vi "Get Result.vi"(8 "error in (no error)":errorcluster, 11 "Addition in":refnum<class "Subtraction.lvclass">) -> (0 "error out":errorcluster, 2 "Result":dbl, 3 "Addition out":refnum<class "Subtraction.lvclass">)   [LabVIEW 2013, in "Operators.lvlib" / "Subtraction.lvclass"]
uses:
  Subtraction.lvclass
  Subtraction.lvclass/Subtraction.ctl
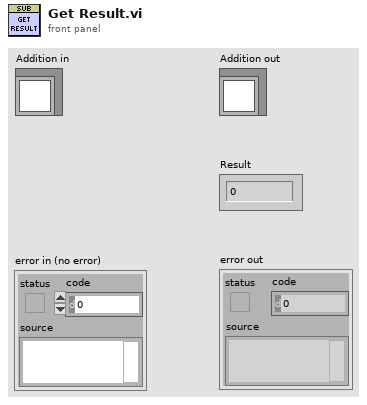
[diagram p1: front panel]
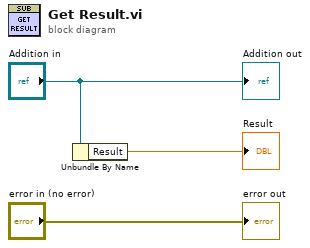
[diagram p0: block diagram]
diagram:
  n1 = Unbundle By Name("Addition in") -> ("Result"=→"Result":dbl)
  "error out" <- "error in (no error)"
  "Addition out" <- "Addition in"
